vi "Set Master Chnls Synch HW.vi"(8 "error in (no error)":errorcluster, 10 "Synch?":bool, 11 "BME_DG_System in":refnum<class "BME_DG_System.lvclass">) -> (0 "error out":errorcluster, 3 "BME_DG_System out":refnum<class "BME_DG_System.lvclass">)   [LabVIEW 2009, in "POLARIS BME DG.lvlib" / "BME_DG_System.lvclass"]
doc: "Sets and Resets Sync Bit at channels of master card. If bit is true, parameter update occurs only if output modulo of channel reaches zero.\n\nlast change:\n20121212 Check if parameter change is still in progress\n\n\nauthor: Alexander Kessler, Helmholtz-Institut-Jena \nmaintainer: Alexander Kessler: alexander.kessler@uni-jena.de\n\nLast Change:\nLicense Agreement for this software:\n\nCopyright (C)\nHelmholtz-Institut-Jena\nFröbelsteg 3\n07743 Jena\nGermany\n\nContact: alexander.kessler@uni-jena.de\n\nThis program is free software; you can redistribute it and/or modify it under the terms of the GNU General Public License as published by the Free Software Foundation; either version 2 of the license, or (at your option) any later version.\n\nThis program is distributed in the hope that it will be useful, but WITHOUT ANY WARRANTY; without even the implied warranty of MERCHANTABILITY or FITNESS FOR A PARTICULAR PURPOSE. See the GNU General License for more details (http://www.gnu.org)."
uses:
  BME_DG_System.lvclass
  BME_DG_Base/BME_DG_Base.lvclass
  LV-BME Interface/GoSignalBits.ctl
  BME_DG_Chnl/BME_DG_Chnl.lvclass
  POLARIS BME DG.lvlib
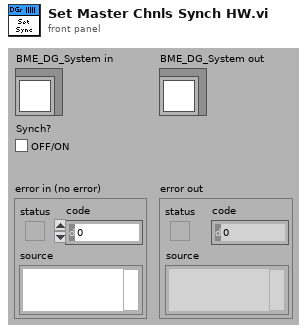
[diagram p1: front panel]
types:
  T1 = typedef "POLARIS BME DG.lvlib/GoSignalBits.ctl" = u32
  T2 = typedef "POLARIS BME DG.lvlib/Chnl Settings Complete.ctl" = cluster{"Channel Name":string, "ChnParameter":T3, "DelayFormula":string, "OutputModulo":i32, "Go and Done Signal":T4, "G08_Chnl_Settings":T5}
  T3 = typedef "POLARIS BME DG.lvlib/ChnlSettings.ctl" = cluster{" Delay (µs)":dbl, "On?":bool, "PositiveVoltage?":bool, "50OhmTerminated? ":bool, "25OhmOutput?":bool}
  T4 = typedef "POLARIS BME DG.lvlib/Go_Done_Chnl_Settings.ctl" = cluster{"Go Signal":T1, "Done Signal":u32}
  T5 = typedef "POLARIS BME DG.lvlib/SG08_Chnl_Settings.ctl" = cluster{"Pulse Width (µs)":dbl, "Output Offset":u32, "Disconnect (E,F)":bool, "Onto MsBus (E,F)":bool, "Input Positive (E,F)":bool}
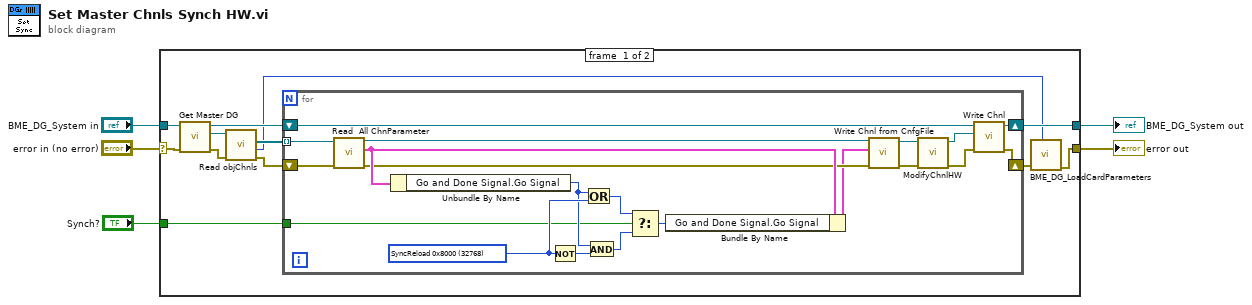
[diagram p0: block diagram]
diagram:
  n1 = case shown="No Error" "error in (no error)" {
    selector: "error in (no error)" -> [w16 w39]
    tunnel: [w7 w39] -> w4
    tunnel: [w9 w38] -> w2
    tunnel: "BME_DG_System in" -> [w17 w38]
    tunnel: "Synch?" -> [w11 _]
    frame #0 {
      n2 = call "Get Master DG.vi"("error in (no error)"=w16, "BME_DG_System in"=w17) -> ("error out"=w14:errorcluster, "BME_DG_Base.lvclass"=w15:refnum<class "BME_DG_Base.lvclass">, "BME_DG_System out"=w10:refnum<class "BME_DG_System.lvclass">)  [unwired: 6 in, 1 out]
      n3 = call-dynamic "Read objChnls.vi"("error in (no error)"=w14, "BME_DG_Base in"=w15) -> ("error out"=w12:errorcluster, "DGNr"=w6:i32, "objChnls"=w13:refnum<class "BME_DG_Chnl.lvclass">[])  [unwired: 6 in, 1 out]
      n4 = for {
        tunnel: w13 -> [w37] mode=indexing
        shift-right: [w18] -> w8
        shift-left: w12 -> [w36]
        tunnel: w11 -> [w31]
        shift-right: [w21] -> w9
        shift-left: w10 -> [w22]
        w34 = T1 32768 items=["Local Primary0x1"=1, "Local Secondary0x2"=2, "Local Force 0x4"=4, "Resynchronize 0x8"=8, "Master Prim. 0x10"=16, "Master Sec. 0x20"=32, "Master Force  0x40"=64, "System Clock 0x80"=128, "Delay Clock 0x100"=256, "Inhibit Local 0x200"=512, "Start Local 0x400"=1024, "Start Bus 0x800"=2048, "Step Back Local 0x1000"=4096, "Step Back Bus 0x2000"=8192, "RunCircle 0x4000"=16384, "SyncReload 0x8000"=32768, "From E 0x10000"=65536, "From F 0x20000"=131072, "From Bus 0x40000"=262144] ("Go and Done Signal.Go Signal")
        n5 = call-dynamic "Read  All ChnParameter.vi"("error in (no error)"=w36, "BME_DG_Chnl in"=w37) -> ("error out"=w27:errorcluster, "ChnlParam"=w35:T2, "BME_DG_Chnl out"=w25:refnum<class "BME_DG_Chnl.lvclass">)  [unwired: 7 in]
        n6 = Unbundle By Name(w35) -> ("Go and Done Signal.Go Signal"=w32:T1)
        n7 = Not(x=w34) -> (.not. x?=w33:T1)
        n8 = Or(x=w32, y=w34) -> (x .or. y?=w30:T1)
        n9 = And(x=w32, y=w33) -> (x .and. y?=w29:T1)
        n10 = Select(t=w30, s=w31, f=w29) -> (s? t:f=w28:T1)
        n11 = Bundle By Name(cluster=w35, "Go and Done Signal.Go Signal"=w28) -> (w24:T2)
        n12 = call-dynamic "Write Chnl from CnfgFile.vi"("error in (no error)"=w27, "ChnlSettings"=w24, "BME_DG_Chnl in"=w25) -> ("error out"=w26:errorcluster, "BME_DG_Chnl out"=w23:refnum<class "BME_DG_Chnl.lvclass">)  [unwired: 7 in]
        n13 = call-dynamic "ModifyChnlHW.vi"("error in (no error)"=w26, "BME_DG_Chnl in"=w23) -> ("error out"=w19:errorcluster, "BME_DG_Chnl out"=w20:refnum<class "BME_DG_Chnl.lvclass">)  [unwired: 8 in]
        n14 = call "Write Chnl.vi"("error in (no error)"=w19, "BME_DG_Chnl.lvclass"=w20, "BME_DG_System in"=w22) -> ("error out"=w18:errorcluster, "BME_DG_System out"=w21:refnum<class "BME_DG_System.lvclass">)  [unwired: 7 in]
      }
      n15 = call "BME_DG_LoadCardParameters.vi"("DG_Number"=w6, "error in (no error)"=w8) -> ("error out"=w7:errorcluster)  [unwired: 9 in]
    }
    frame #1 {
    }
  }
  "error out" <- w4
  "BME_DG_System out" <- w2
